vi "Shifter.vi"() -> ()   [LabVIEW 2011]
uses:
  <vilib>/Rock Robotics/WPI/Solenoid/WPI_SolenoidDevRef.ctl
  <vilib>/Rock Robotics/SystemInterfaces/Typedef/FPGA_TypedefSolenoidModule.ctl
  <vilib>/Rock Robotics/WPI/Solenoid/WPI_SolenoidChannel.ctl
  <vilib>/Rock Robotics/WPI/Solenoid/WPI_SolenoidValue.ctl
  <vilib>/Rock Robotics/WPI/Solenoid/WPI_SolenoidGetEnum.vi
  <vilib>/Rock Robotics/WPI/Solenoid/WPI_SolenoidSetEnum.vi
panel:
  in  "Right Shifter":T1={"DevStatus"={"status"=FALSE, "code"=0, "source"=""}, "Solenoid Module"=enum."Solenoid Module 1", "Forward Solenoid Channel"=enum."Invalid", "Reverse Solenoid Channel"=enum."Invalid"}
  in  "Left Shifter":T1={"DevStatus"={"status"=FALSE, "code"=0, "source"=""}, "Solenoid Module"=enum."Solenoid Module 1", "Forward Solenoid Channel"=enum."Invalid", "Reverse Solenoid Channel"=enum."Invalid"}
  in  "Forced High (override)":bool=TRUE
  in  "Shift":bool=TRUE
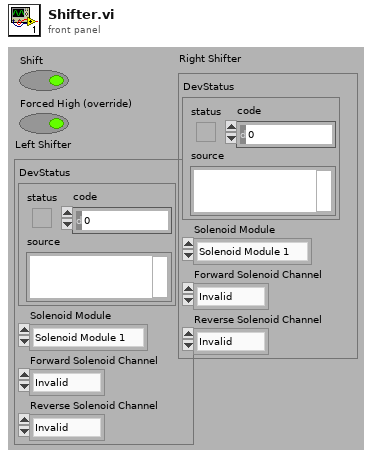
[diagram p1: front panel]
types:
  T1 = typedef "WPI_SolenoidDevRef.ctl" = cluster{"DevStatus":errorcluster, "Solenoid Module":T2, "Forward Solenoid Channel":T3, "Reverse Solenoid Channel":T3}
  T2 = typedef "FPGA_TypedefSolenoidModule.ctl" = enum16{"Solenoid Module 1", "Solenoid Module 2"}
  T3 = typedef "WPI_SolenoidChannel.ctl" = enum8{"Solenoid 1", "Solenoid 2", "Solenoid 3", "Solenoid 4", "Solenoid 5", "Solenoid 6", "Solenoid 7", "Solenoid 8", "Invalid"}
  T4 = typedef "WPI_SolenoidValue.ctl" = enum16{"Off", "On", "Forward", "Reverse"}
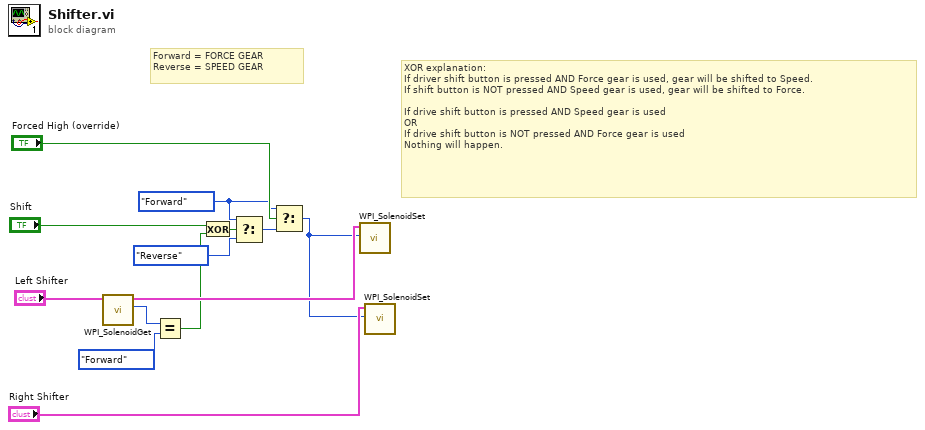
[diagram p0: block diagram]
diagram:
  w2 = WPI_SolenoidValue."Forward" ("Value")
  # "XOR explanation:\nIf driver shift button is pressed AND Force gear is used, gear will be shifted to Speed.\nIf shift button is NOT pressed AND Speed gear is used, gear will be shifted to Force.\n\nIf drive shift button is pressed AND Speed gear is used\nOR\nIf drive shift button is NOT pressed AND Force gear is used\nNothing will happen."
  # "Forward = FORCE GEAR\nReverse = SPEED GEAR"
  n1 = call-poly <vilib>:"WPI_SolenoidGet.vi"("SolenoidDevRef"="Left Shifter") -> ("Value"=w10:T4, "SolenoidDevRef"=w11:T1)  [unwired: 1 in, 8 out]
  n2 = Equal?(x=w10, y=WPI_SolenoidValue."Forward" ("Value")) -> (x = y?=w8:bool)
  n3 = Exclusive Or(1:w8, 2:"Shift") -> (0:w6:bool)
  n4 = Select(t=w2, s=w6, f=WPI_SolenoidValue."Reverse" ("Value")) -> (s? t:f=w4:T4)
  n5 = Select(t=w2, s="Forced High (override)", f=w4) -> (s? t:f=w1:T4)
  n6 = call-poly <vilib>:"WPI_SolenoidSet.vi"("Value"=w1, "SolenoidDevRef"=w11) -> ()  [unwired: 1 in, 9 out]
  n7 = call-poly <vilib>:"WPI_SolenoidSet.vi"("Value"=w1, "SolenoidDevRef"="Right Shifter") -> ()  [unwired: 1 in, 9 out]
